vi "MGI Match String in Element.vi"(5 "Precedence (Index)":T1, 7 "Match Pattern? (F)":bool, 9 "Match":string, 11 "String[]":string[](array[string])) -> (1 "Index":i32, 2 "Offset past match":i32, 3 "Match":string)   [LabVIEW 2016]
doc: "This VI searches each element of<B>String[]</B> for an occurence of <B>Match</B>. If no match is found, then <B>Offset past match</B> and <B>Index</B> are -1, and <B>Match</B> is empty.\n<B>Precedence</B> determines result if multple matches exist. For example:\nString[]={\"AB\",\"BC\"}\nMatch[] = \"B\"\nIf <B>Precedence</B> is <B>Index</B>, then Index is 0. If it is <B>Offset</B>, then Index is 1.\n\nAuthored by Shawn Walpole\nsupport@mooregoodideas.com\nwww.mooregoodideas.com\n\nCopyright (c) 2010, Moore Good Ideas, Inc.\n\nAll rights reserved.\n\nRedistribution and use in source and binary forms, with or without modification, are permitted provided that the following conditions are met:\n\n * Redistributions of source code must retain the above copyright notice, this list of conditions and the following disclaimer.\n * Redistributions in binary form must reproduce the above copyright notice, this list of conditions and the following disclaimer in the documentation and/or other materials provided with the distribution.\n * Neither the name of Moore Good Ideas, Inc. nor the names of its contributors may be used to endorse or promote products derived from this software without specific prior written permission.\n\nTHIS SOFTWARE IS PROVIDED BY THE COPYRIGHT HOLDERS AND CONTRIBUTORS \"AS IS\" AND ANY EXPRESS OR IMPLIED WARRANTIES, INCLUDING, BUT NOT LIMITED TO, THE IMPLIED WARRANTIES OF MERCHANTABILITY AND FITNESS FOR A PARTICULAR PURPOSE ARE DISCLAIMED. IN NO EVENT SHALL THE COPYRIGHT OWNER OR CONTRIBUTORS BE LIABLE FOR ANY DIRECT, INDIRECT, INCIDENTAL, SPECIAL, EXEMPLARY, OR CONSEQUENTIAL DAMAGES (INCLUDING, BUT NOT LIMITED TO, PROCUREMENT OF SUBSTITUTE GOODS OR SERVICES; LOSS OF USE, DATA, OR PROFITS; OR BUSINESS INTERRUPTION) HOWEVER CAUSED AND ON ANY THEORY OF LIABILITY, WHETHER IN CONTRACT, STRICT LIABILITY, OR TORT (INCLUDING NEGLIGENCE OR OTHERWISE) ARISING IN ANY WAY OUT OF THE USE OF THIS SOFTWARE, EVEN IF ADVISED OF THE POSSIBILITY OF SUCH DAMAGE."
uses:
  <userlib>/_MGI/String/MGI Match Precedence Enum.ctl
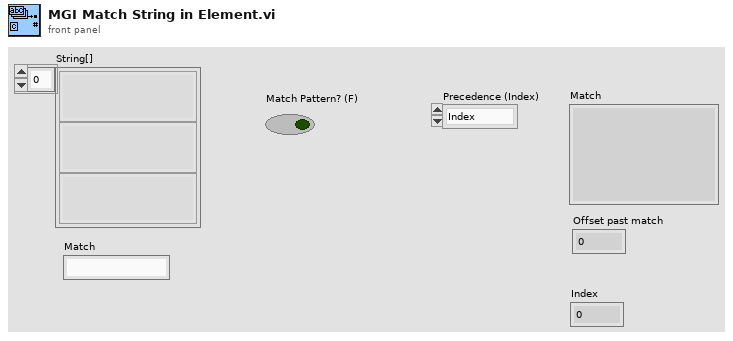
[diagram p1: front panel]
types:
  T1 = typedef "MGI Match Precedence Enum.ctl" = enum16{"Index", "Offset"}
  T2 = cluster{"offset past match":i32, "offset past match":i32, i32, "Match":string}
  T3 = cluster{"offset past match":i32, "offset past match":i32, i32, "Match":string}[]
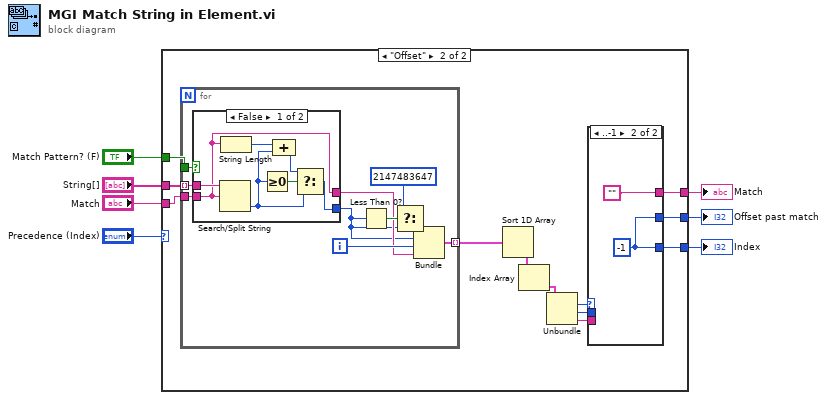
[diagram p0: block diagram]
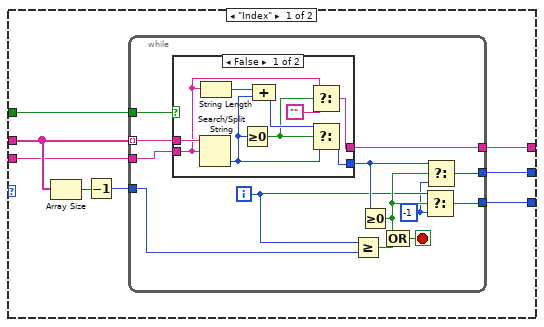
[diagram p2: hidden frame]
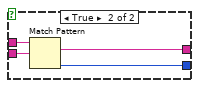
[diagram p3: hidden frame]
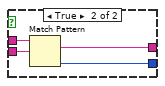
[diagram p5: hidden frame]
diagram:
  n1 = case shown="\"Offset\"" "Precedence (Index)" {
    tunnel: "Match" -> [w14 w53]
    tunnel: [w9 w52] -> w2
    tunnel: "String[]" -> [w15 w51]
    tunnel: [w11 w50] -> w4
    tunnel: [w10 w49] -> w3
    tunnel: "Match Pattern? (F)" -> [w8 w42]
    frame "Index" {
      n2 = Array Size(array=w15) -> (size(s)=w13:i32)
      n3 = Decrement(x=w13) -> (x-1=w12:i32)
      n4 = while {
        tunnel: w14 -> [w18]
        tunnel: w15 -> [w17] mode=indexing
        tunnel: w12 -> [w28]
        tunnel: [w25] -> w11
        tunnel: [w22] -> w10
        tunnel: [w20] -> w9
        tunnel: w8 -> [w19]
        i -> [w21]
        stop <- w26 stop-if-true
        w16 = -1 ("f")
        n5 = case shown="False" w19 {
          tunnel: w17 -> [w37 w41]
          tunnel: w18 -> [w31 w40]
          tunnel: [w29 w39] -> w25
          tunnel: [w34 w38] -> w23
          frame False {
            n6 = Search/Split String(string=w37, search string/char (-)=w31) -> (offset of match=w33:i32)  [unwired: 1 in, 2 out]
            n7 = String Length(string=w31) -> (length=w36:i32)
            n8 = Greater Or Equal To 0?(x=w33) -> (x >= 0?=w32:bool)
            n9 = Compound Arithmetic op=ADD(w36, w33) -> (w35:i32)
            n10 = Select(t=w31, s=w32, f="") -> (s? t:f=w29:string)
            n11 = Select(t=w35, s=w32, f=w33) -> (s? t:f=w34:i32)
          }
          frame True {
            n12 = Match Pattern(string=w41, regular expression=w40) -> (match substring=w39:string, offset past match=w38:i32)  [unwired: 1 in, 2 out]
          }
        }
        n13 = Greater Or Equal?(x=w21, y=w28) -> (x >= y?=w27:bool)
        n14 = Greater Or Equal To 0?(x=w23) -> (x >= 0?=w24:bool)
        n15 = Compound Arithmetic op=OR(w24, w27) -> (w26:bool)
        n16 = Select(t=w21, s=w24, f=w16) -> (s? t:f=w20:i32)
        n17 = Select(t=w23, s=w24, f=w16) -> (s? t:f=w22:i32)
      }
    }
    frame "Offset" {
      n18 = for {
        tunnel: w51 -> [w62] mode=indexing
        tunnel: [w64] -> w48 mode=indexing
        tunnel: w53 -> [w61]
        tunnel: w42 -> [w63]
        i -> [w65]
        n19 = case shown="False" w63 {
          tunnel: w62 -> [w75 w79]
          tunnel: w61 -> [w74 w78]
          tunnel: [w74 w77] -> w60
          tunnel: [w71 w76] -> w59
          frame False {
            n20 = Search/Split String(string=w75, search string/char (-)=w74) -> (offset of match=w69:i32)  [unwired: 1 in, 2 out]
            n21 = String Length(string=w74) -> (length=w73:i32)
            n22 = Greater Or Equal To 0?(x=w69) -> (x >= 0?=w70:bool)
            n23 = Compound Arithmetic op=ADD(w73, w69) -> (w72:i32)
            n24 = Select(t=w72, s=w70, f=w69) -> (s? t:f=w71:i32)
          }
          frame True {
            n25 = Match Pattern(string=w79, regular expression=w78) -> (match substring=w77:string, offset past match=w76:i32)  [unwired: 1 in, 2 out]
          }
        }
        n26 = Less Than 0?(x=w59) -> (x < 0?=w68:bool)
        n27 = Select(t=2147483647 ("f"), s=w68, f=w59) -> (s? t:f=w66:i32)
        n28 = Bundle("offset past match"=w66, "offset past match"=w59, w65, "Match"=w60) -> (w64:T2)  [unwired: 1 in]
      }
      n29 = Sort 1D Array(array=w48) -> (sorted array=w47:T3)
      n30 = Index Array(array=w47) -> (element=w46:T2)  [unwired: 1 in]
      n31 = Unbundle(w46) -> ("offset past match"=w45:i32, w43:i32, "Match"=w44:string)  [unwired: 1 out]
      n32 = case shown="..-1" w45 {
        selector: w45 -> [w56 _]
        tunnel: [w56 w57] -> w49
        tunnel: [w55 ""] -> w50
        tunnel: [w54 w57] -> w52
        tunnel: w44 -> [w55 _]
        tunnel: w43 -> [w54 _]
        frame 0.. {
        }
        frame ..-1 {
          w57 = -1 ("f")
        }
      }
    }
  }
  "Offset past match" <- w3
  "Index" <- w2
  "Match" <- w4
